vi "QCA Generate Event.vi"(0 "Event Number":i32) -> ()   [LabVIEW 2019]
uses:
  QCA Global.vi
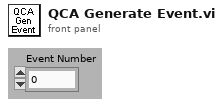
[diagram p1: front panel]
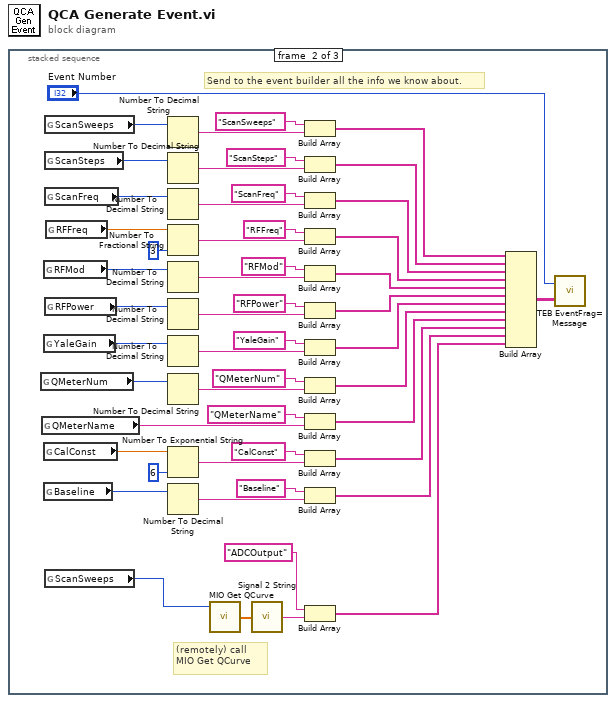
[diagram p0: block diagram]
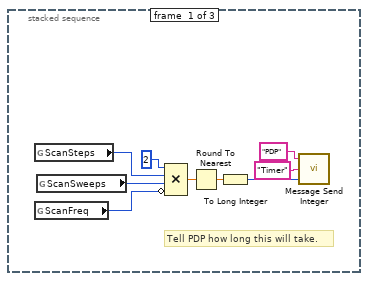
[diagram p2: hidden frame]
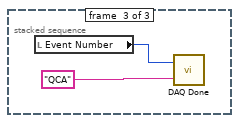
[diagram p3: hidden frame]
diagram:
  n1 = stacked-sequence {
    frame #0 {
      # "Tell PDP how long this will take."
      n2 = global read "QCA Global.vi" "ScanSteps"() -> (w2:i32)
      n3 = global read "QCA Global.vi" "ScanFreq"() -> (w4:i32)
      n4 = global read "QCA Global.vi" "ScanSweeps"() -> (w1:i32)
      n5 = Compound Arithmetic op=MULTIPLY(2 ("Input"), w2, w1, invert w4) -> (w5:dbl)
      n6 = Round To Nearest(number=w5) -> (nearest integer value=w6:dbl)
      n7 = To Long Integer(number=w6) -> (32bit integer=w9:i32)
      n8 = call "Message Send Integer.vi"("Value"=w9, "Parameter"="Timer", "Destination"="PDP") -> ()
    }
    frame #1 {
      # "(remotely) call MIO Get QCurve"
      # "Send to the event builder all the info we know about."
      n9 = global read "QCA Global.vi" "QMeterNum"() -> (w19:i32)
      n10 = global read "QCA Global.vi" "QMeterName"() -> (w32:string)
      n11 = global read "QCA Global.vi" "RFMod"() -> (w48:i32)
      n12 = global read "QCA Global.vi" "YaleGain"() -> (w42:i32)
      n13 = global read "QCA Global.vi" "CalConst"() -> (w38:dbl)
      n14 = global read "QCA Global.vi" "Baseline"() -> (w33:i32)
      n15 = global read "QCA Global.vi" "ScanSweeps"() -> (w60:i32)
      n16 = global read "QCA Global.vi" "ScanSteps"() -> (w55:i32)
      n17 = global read "QCA Global.vi" "ScanFreq"() -> (w54:i32)
      n18 = global read "QCA Global.vi" "RFPower"() -> (w43:i32)
      n19 = global read "QCA Global.vi" "ScanSweeps"() -> (w10:i32)
      n20 = global read "QCA Global.vi" "RFFreq"() -> (w49:dbl)
      n21 = Number To Decimal String(number=w60) -> (decimal integer string=w59:string)  [unwired: 1 in]
      n22 = Number To Decimal String(number=w55) -> (decimal integer string=w56:string)  [unwired: 1 in]
      n23 = Number To Decimal String(number=w54) -> (decimal integer string=w53:string)  [unwired: 1 in]
      n24 = Number To Fractional String(number=w49, precision (6)=i16 3) -> (F-format string=w50:string)  [unwired: 2 in]
      n25 = Number To Decimal String(number=w48) -> (decimal integer string=w47:string)  [unwired: 1 in]
      n26 = Number To Decimal String(number=w43) -> (decimal integer string=w44:string)  [unwired: 1 in]
      n27 = Number To Decimal String(number=w42) -> (decimal integer string=w41:string)  [unwired: 1 in]
      n28 = Number To Decimal String(number=w19) -> (decimal integer string=w20:string)  [unwired: 1 in]
      n29 = Number To Exponential String(number=w38, precision (6)=i16 6) -> (E-format string=w37:string)  [unwired: 2 in]
      n30 = Number To Decimal String(number=w33) -> (decimal integer string=w34:string)  [unwired: 1 in]
      n31 = call "MIO Get QCurve.vi"("Num Sweeps"=w10) -> ("Waveform Graph"=w11:dbl[])  [unwired: 2 in]
      n32 = call "Signal 2 String.vi"("Signal"=w11) -> ("String"=w12:string)
      n33 = Build Array("ScanSweeps" ("Substring"), w59) -> (w29:string[])
      n34 = Build Array("ScanSteps" ("Substring"), w56) -> (w28:string[])
      n35 = Build Array("ScanFreq" ("Substring"), w53) -> (w27:string[])
      n36 = Build Array("RFFreq" ("Substring"), w50) -> (w26:string[])
      n37 = Build Array("RFMod" ("Substring"), w47) -> (w23:string[])
      n38 = Build Array("RFPower" ("Substring"), w44) -> (w24:string[])
      n39 = Build Array("YaleGain" ("Substring"), w41) -> (w25:string[])
      n40 = Build Array("QMeterNum" ("Substring"), w20) -> (w15:string[])
      n41 = Build Array("QMeterName" ("Substring"), w32) -> (w16:string[])
      n42 = Build Array("CalConst" ("Substring"), w37) -> (w17:string[])
      n43 = Build Array("Baseline" ("Substring"), w34) -> (w18:string[])
      n44 = Build Array("ADCOutput", w12) -> (w14:string[])
      n45 = Build Array(w29, w28, w27, w26, w23, w24, w25, w15, w16, w17, w18, w14) -> (w22:string[][])
      n46 = call "TEB EventFrag= Message.vi"("Event Fragment(s)"=w22, "Event Number"="Event Number") -> ()
    }
    frame #2 {
      n47 = local read "Event Number"() -> (w63:i32)
      n48 = call "DAQ Done.vi"("Module Name"="QCA", "Event Number"=w63) -> ()
    }
  }
